vi "Grid Direction Position.vi"(10 "Direction":T2, 11 "From":T1) -> (2 "Opposite":T2, 3 "To":T1)   [LabVIEW 2020, in "Maze.lvlib"]
uses:
  Maze.lvlib
  Position.ctl
  Direction.ctl
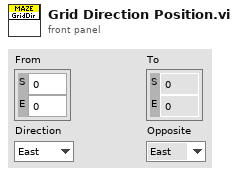
[diagram p1: front panel]
types:
  T1 = typedef "Maze.lvlib/Position.ctl" = cluster{"S":i32, "E":i32}
  T2 = typedef "Maze.lvlib/Direction.ctl" = enum8{"East", "North", "West", "South"}
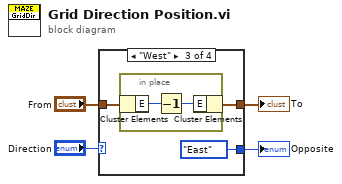
[diagram p0: block diagram]
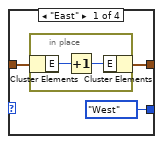
[diagram p2: hidden frame]
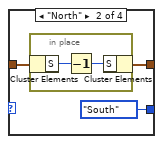
[diagram p3: hidden frame]
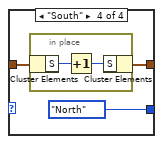
[diagram p4: hidden frame]
diagram:
  n1 = case shown="\"West\"" "Direction" {
    tunnel: "From" -> [w7 w12 w17 w22]
    tunnel: [w6 w11 w16 w21] -> w2
    tunnel: [Direction."West" ("Opposite") Direction."South" ("Opposite") Direction."East" ("Opposite") Direction."North" ("Opposite")] -> w1
    frame "East" {
      n2 = in-place {
        n3 = in-place-cluster #1(w7) -> ("E"=w9:i32)
        n4 = Increment(x=w9) -> (x+1=w8:i32)
        n5 = in-place-cluster #1("E"=w8) -> (w6:T1)
      }
    }
    frame "North" {
      n6 = in-place {
        n7 = in-place-cluster #2(w12) -> ("S"=w14:i32)
        n8 = Decrement(x=w14) -> (x-1=w13:i32)
        n9 = in-place-cluster #2("S"=w13) -> (w11:T1)
      }
    }
    frame "West" {
      n10 = in-place {
        n11 = in-place-cluster #3(w17) -> ("E"=w19:i32)
        n12 = Decrement(x=w19) -> (x-1=w18:i32)
        n13 = in-place-cluster #3("E"=w18) -> (w16:T1)
      }
    }
    frame "South" {
      n14 = in-place {
        n15 = in-place-cluster #4(w22) -> ("S"=w24:i32)
        n16 = Increment(x=w24) -> (x+1=w23:i32)
        n17 = in-place-cluster #4("S"=w23) -> (w21:T1)
      }
    }
  }
  "Opposite" <- w1
  "To" <- w2
